vi "Monitor Data Changed.vi"(8 "error in (no error)":errorcluster, 9 "Changed Actor Q":refnum<class "Message Enqueuer.lvclass">, 10 "Monitor Data":refnum<class "Monitor Data.lvclass">, 11 "Classic Actor Monitor in":refnum<class "Classic Monitor.lvclass">) -> (0 "error out":errorcluster, 3 "Classic Actor Monitor out":refnum<class "Classic Monitor.lvclass">)   [LabVIEW 2023, in "Monitored Actor.lvlib" / "Classic Monitor.lvclass"]
doc: "Messages the UI with the new Monitor Data\n\nCopyright: MGI 2016\nAuthor: Derek Trepanier"
uses:
  Classic Monitor.lvclass
  Monitor Data/Monitor Data.lvclass
  builds/Framework/Actor Framework.lvlibp/1abvi3w/vi.lib/ActorFramework/Message Enqueuer/Message Enqueuer.lvclass
  Classic Monitor.lvclass/Classic Monitor.ctl
  Orphan Detector/Orphan Detector Messages/Monitor Stop Msg/Monitor Stop Msg.lvclass
  Logger/Classic Logger Messages/Update Monitor Label Msg/Update Monitor Label Msg.lvclass
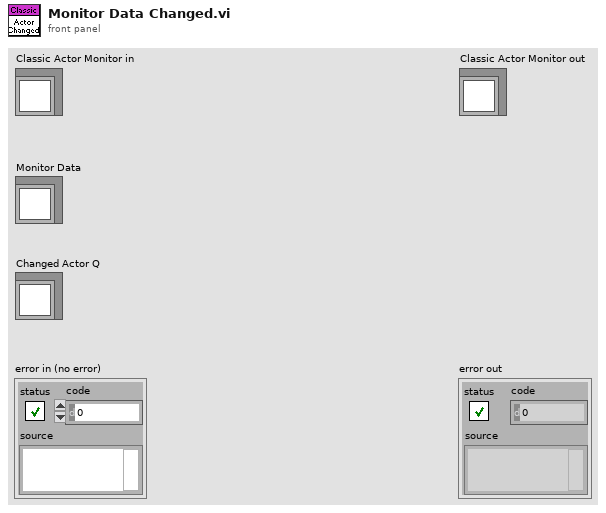
[diagram p1: front panel]
types:
  T1 = typedef "Monitored Actor.lvlib/Monitor Data.lvclass/Actor Data.ctl" = cluster{"Actor Type":string, "Actor Core VI":string, "Self":refnum<class "Message Enqueuer.lvclass">, "Caller":refnum<class "Message Enqueuer.lvclass">, "Actor Label":string, "Last Ping":dbl}
  T2 = cluster{"Monitor Data":refnum<class "Monitor Data.lvclass">, "Changed Actor Q":refnum<class "Message Enqueuer.lvclass">}
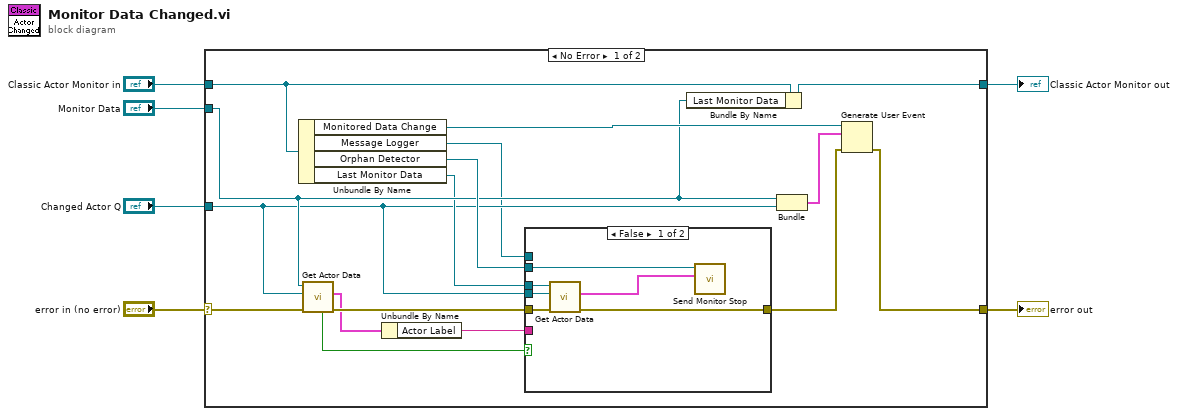
[diagram p0: block diagram]
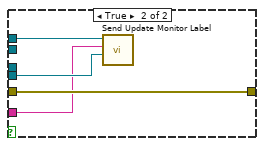
[diagram p2: hidden frame]
diagram:
  n1 = case shown="No Error" "error in (no error)" {
    selector: "error in (no error)" -> [w18 w33]
    tunnel: [w20 w33] -> w6
    tunnel: [w13 w34] -> w5
    tunnel: "Monitor Data" -> [w12 _]
    tunnel: "Classic Actor Monitor in" -> [w22 w34]
    tunnel: "Changed Actor Q" -> [w10 _]
    frame No Error {
      n2 = Unbundle By Name(w22) -> ("Monitored Data Change"=w21:refnum<user-event>, "Message Logger"=w9:refnum<class "Message Enqueuer.lvclass">, "Orphan Detector"=w17:refnum<class "Message Enqueuer.lvclass">, "Last Monitor Data"=w11:refnum<class "Monitor Data.lvclass">)
      n3 = call "Get Actor Data.vi"("error in (no error)"=w18, "Actor's Self Q"=w10, "Monitor Data in"=w12) -> ("error out"=w16:errorcluster, "Actor Data"=w8:T1, "Found?"=w14:bool)  [unwired: 4 in, 2 out]
      n4 = Unbundle By Name(w8) -> ("Actor Label"=w7:string)
      n5 = case shown="False" w14 {
        tunnel: w17 -> [w28 _]
        tunnel: w16 -> [w27 w32]
        tunnel: [w23 w32] -> w15
        tunnel: w11 -> [w25 _]
        tunnel: w10 -> [w24 w30]
        tunnel: w9 -> [_ w31]
        tunnel: w7 -> [_ w29]
        frame False {
          n6 = call "Get Actor Data.vi"("error in (no error)"=w27, "Actor's Self Q"=w24, "Monitor Data in"=w25) -> ("error out"=w23:errorcluster, "Actor Data"=w26:T1)  [unwired: 4 in, 3 out]
          n7 = call "Send Monitor Stop.vi"("Actor Data"=w26, "Message Enqueuer in"=w28) -> ()  [unwired: 8 in, 2 out]
        }
        frame True {
          n8 = call "Send Update Monitor Label.vi"("Actor to Log"=w30, "Label"=w29, "Message Enqueuer in"=w31) -> ()  [unwired: 7 in, 2 out]
        }
      }
      n9 = Bundle By Name(cluster=w22, "Last Monitor Data"=w12) -> (w13:refnum<class "Classic Monitor.lvclass">)
      n10 = Bundle("Monitor Data"=w12, "Changed Actor Q"=w10) -> (w19:T2)  [unwired: 1 in]
      n11 = Generate User Event(user event=w21, event data cluster=w19, error in=w15) -> (error out=w20:errorcluster)  [unwired: 1 in, 1 out]
    }
    frame Error {
    }
  }
  "error out" <- w6
  "Classic Actor Monitor out" <- w5
